vi "everyn.vi"() -> ()   [LabVIEW 2021]
uses:
  <vilib>/numeric/Random Number (Range) I64.vi
  d961f8f4-1d9d-44d3-84fb-bd166e71486c.vi
  <vilib>/numeric/sub_Random U32.vi
  <vilib>/Comparison/Less/Less Functor/Less Functor.lvclass
panel:
  out "appended array":i64[](array[numeric])
  out "sorted array":i64[](array[numeric])
  out "multiply every n":i64
  out "XY Graph":cluster{i32[], i64[]}(graph)
  out "random array":i64[](array[numeric])
  in  "enter T (massive lenghts)":dbl
  in  "enter n":dbl
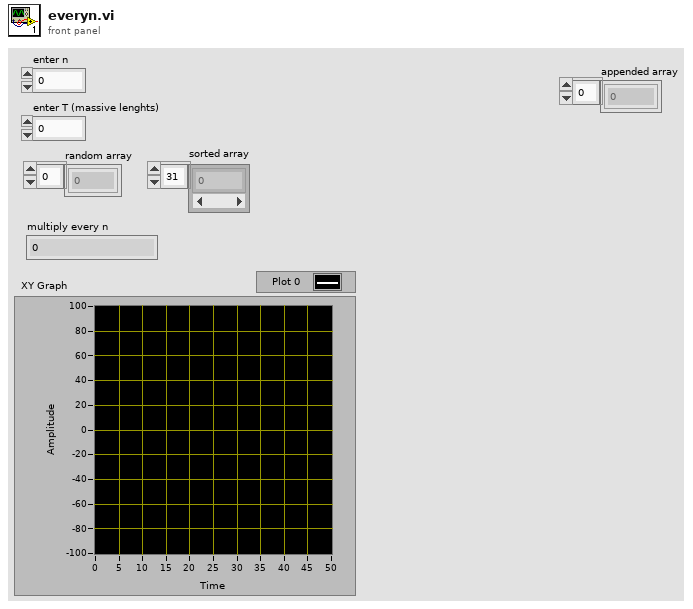
[diagram p1: front panel]
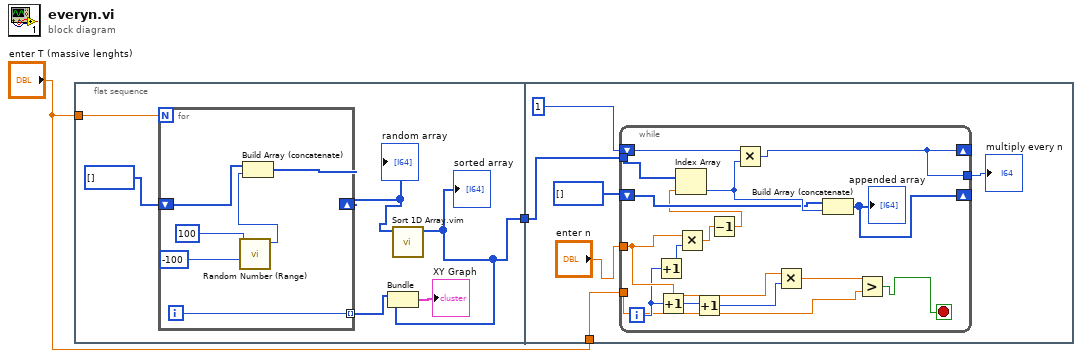
[diagram p0: block diagram]
diagram:
  n1 = flat-sequence {
    tunnel: "enter T (massive lenghts)" -> [w4]
    tunnel: [w3] -> w2
    tunnel: w2 -> [w19]
    tunnel: "enter T (massive lenghts)" -> [w18]
    frame #0 {
      n2 = for {
        N: w4 -> [_]
        shift-right: [w10] -> w5
        shift-left: i32[] [] -> [w12]
        tunnel: [w9] -> w6 mode=indexing
        i -> [w9]
        n3 = call-poly <vilib>:"Random Number (Range).vi"("lower bound (-100)"=i64 -100 ("lower bound (0)"), "upper bound (100)"=i64 100) -> ("number"=w11:i64)  [unwired: 9 in]
        n4 = Build Array (concatenate)(w12, w11) -> (w10:i64[])
      }
      "random array" <- w5
      n5 = call "Sort 1D Array.vim"("unsorted array"=w5) -> ("sorted array"=w3:i64[])  [unwired: 10 in]
      "sorted array" <- w3
      n6 = Bundle(w6, "sorted array"=w3) -> (→"XY Graph":cluster{i32[], "sorted array":i64[]})  [unwired: 1 in]
    }
    frame #1 {
      n7 = while {
        tunnel: w19 -> [w36]
        shift-right: [w34] -> _
        shift-left: 1 -> [w35]
        tunnel: [w34] -> w20
        tunnel: w18 -> [w22]
        shift-right: [w31] -> _
        shift-left: i32[] [] -> [w32]
        tunnel: "enter n" -> [w27]
        i -> [w25]
        stop <- w23 stop-if-true
        n8 = Increment(x=w25) -> (x+1=w29:i32)
        n9 = Increment(x=w25) -> (x+1=w26:i32)
        n10 = Multiply(x=w27, y=w29) -> (x*y=w28:dbl)
        n11 = Increment(x=w26) -> (x+1=w24:i32)
        n12 = Decrement(x=w28) -> (x-1=w30:dbl)
        n13 = Index Array(array=w36, index=w30) -> (element=w33:i64)
        n14 = Multiply(x=w35, y=w33) -> (x*y=w34:i64)
        n15 = Multiply(x=w27, y=w24) -> (x*y=w21:dbl)
        n16 = Build Array (concatenate)(w32, w33) -> (w31:i64[])
        "appended array" <- w31
        n17 = Greater?(x=w21, y=w22) -> (0:w23:bool)
      }
      "multiply every n" <- w20
    }
  }
